vi "Popup Long Integer.vi"(8 "error in (no error)":errorcluster, 9 "Panel":refnum<class "Panel.lvclass">, 10 "String in":string, 11 "Numeric Data Type in":refnum<class "Numeric Data Type.lvclass">) -> (0 "error out":errorcluster, 2 "String out":string, 3 "Numeric Data Type out":refnum<class "Numeric Data Type.lvclass">)   [LabVIEW 2018, in "Numeric Data Type.lvclass"]
uses:
  Numeric Data Type.lvclass
  <vilib>/MGI/Panel Manager/Panel/Panel/Panel.lvclass
  Numeric Data Type.lvclass/Numeric Data Type.ctl
  <vilib>/Utility/miscctls.llb/LVPointTypeDef.ctl
panel:
  in  "Numeric":i32
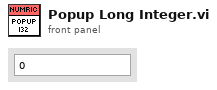
[diagram p1: front panel]
types:
  T1 = typedef "Numeric Data Type.lvclass/Response to Values Outside of Limits Enum.ctl" = enum16{"Ignore", "Coerce to nearest", "Coerce up", "Coerce down"}
  T2 = typedef "LVPointTypeDef.ctl" = cluster{"Horizontal":i16, "Vertical":i16}
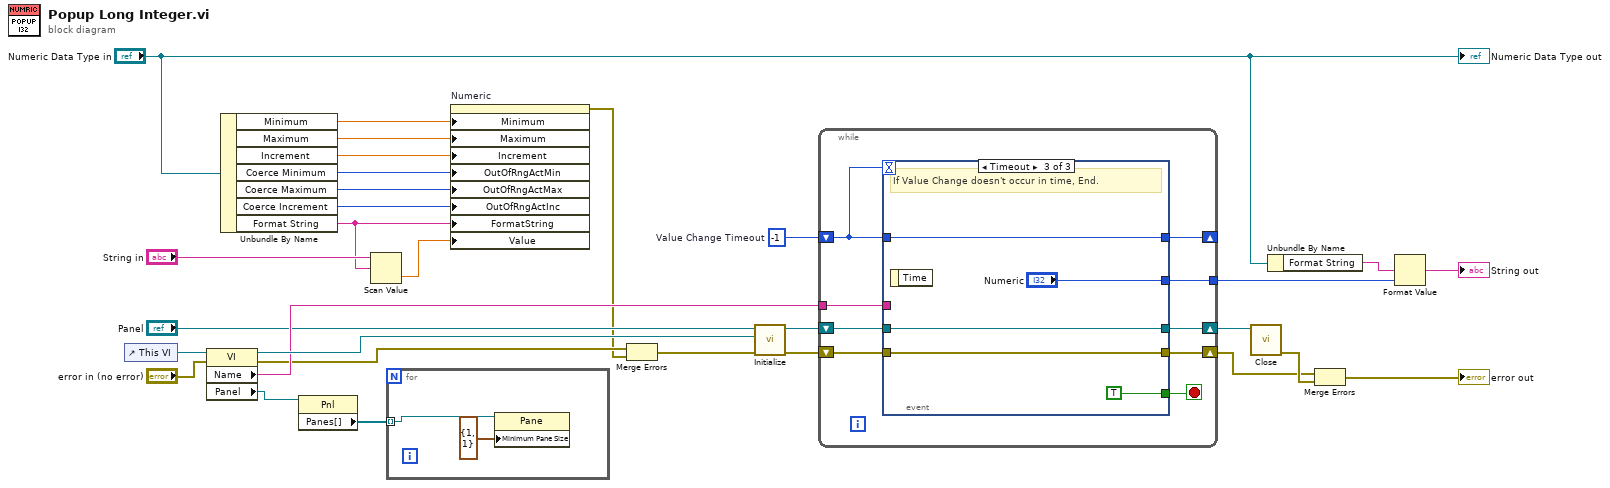
[diagram p0: block diagram]
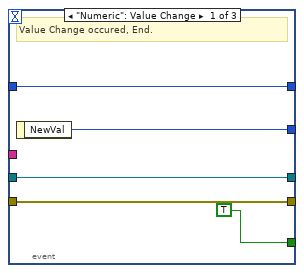
[diagram p2: hidden frame]
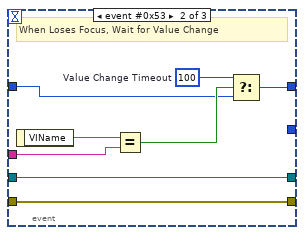
[diagram p3: hidden frame]
diagram:
  w30 = -1  # Value Change Timeout
  n1 = control-ref of="This VI"() -> (w27:refnum<vi>)
  n2 = property class="VI"(reference=w27, error in="error in (no error)") -> (reference out=w26:refnum<vi>, error out=w18:errorcluster, "Name"=w25:string, "Panel"=w2:refnum<vi>)
  n3 = Unbundle By Name("Numeric Data Type in") -> ("Minimum"=w16:dbl, "Maximum"=w15:dbl, "Increment"=w14:dbl, "Coerce Minimum"=w13:T1, "Coerce Maximum"=w12:T1, "Coerce Increment"=w11:T1, "Format String"=w10:string)
  n4 = property class="Pnl"(reference=w2) -> ("Panes[]"=w1:refnum<vi>[])  [unwired: 1 in, 2 out]
  n5 = Scan Value(string="String in", format string=w10) -> (value=w9:dbl)  [unwired: 1 in, 1 out]
  n6 = for {
    tunnel: w1 -> [w32] mode=indexing
    n7 = property class="Pane"(reference=w32, "Minimum Pane Size"=T2 {"Horizontal"=1, "Vertical"=1}) -> ()  [unwired: 1 in, 2 out]
  }
  n8 = property on="Numeric" class="DigNum (strict)"("Minimum"=w16, "Maximum"=w15, "Increment"=w14, "OutOfRngActMin"=w13, "OutOfRngActMax"=w12, "OutOfRngActInc"=w11, "FormatString"=w10, "Value"=w9) -> (error out=w7:errorcluster)  [unwired: 2 in, 1 out]
  n9 = Merge Errors(w18, w7) -> (w8:errorcluster)
  n10 = call <vilib>:"Initialize.vi"("error in (no error)"=w8, "VI Refnum"=w26, "Panel In"="Panel") -> ("error out"=w28:errorcluster, "Panel Out"=w29:refnum<class "Panel.lvclass">)  [unwired: 6 in, 1 out]
  n11 = while {
    shift-right: [w41] -> w22
    shift-left: w28 -> [w40]
    shift-right: [w38] -> w23
    shift-left: w29 -> [w37]
    tunnel: [w36] -> w6
    tunnel: w25 -> [w35]
    shift-right: [w33] -> _
    shift-left: w30 -> [w34]
    stop <- w39 stop-if-true
    n12 = event shown="[2] Timeout" {
      selector: _ -> [_ _ _]
      dyn-events: _ -> [_ _ _]
      timeout: w34 -> [_ _ _]
      tunnel: [w43 w52 w57] -> w41
      tunnel: w40 -> [w43 w52 w57]
      tunnel: [TRUE _ TRUE] -> w39
      tunnel: [w45 w51 w58] -> w38
      tunnel: w37 -> [w45 w51 w58]
      tunnel: [w44 _ "Numeric"] -> w36
      tunnel: w35 -> [_ w53 _]
      tunnel: w34 -> [w42 w48 w55]
      tunnel: [w42 w47 w55] -> w33
      event "Numeric": Value Change {
        # "Value Change occured, End."
        n13 = event-data() -> ("NewVal"=w44:i32)  [unwired: 1 in]
      }
      event event #0x53 {
        w49 = 100  # Value Change Timeout
        # "When Loses Focus, Wait for Value Change"
        n14 = event-data() -> ("VIName"=w54:string)  [unwired: 1 in]
        n15 = Equal?(x=w54, y=w53) -> (x = y?=w50:bool)
        n16 = Select(t=w49, s=w50, f=w48) -> (s? t:f=w47:i32)
      }
      event Timeout {
        # "If Value Change doesn't occur in time, End."
        n17 = event-data() -> ()  [unwired: 1 in, 1 out]
      }
    }
  }
  n18 = call-dynamic "Close.vi"("Panel In"=w23) -> ("Error Out"=w24:errorcluster)  [unwired: 10 in]
  n19 = Unbundle By Name("Numeric Data Type in") -> ("Format String"=w4:string)
  n20 = Merge Errors(w22, w24) -> (→"error out":errorcluster)
  n21 = Format Value(format string=w4, value (0)=w6) -> (output string=→"String out":string)  [unwired: 1 in]
  "Numeric Data Type out" <- "Numeric Data Type in"
